vi "AC Couple (1 Ch DBL Array).vi"(8 "error in (no error)":errorcluster, 10 "Signal":dbl[](array[numeric])) -> (0 "error out":errorcluster, 1 "DC":dbl, 2 "AC Coupled":dbl[](array[numeric]))   [LabVIEW 2017, in "VibrationAnalysisFunctions.lvlib"]
uses:
  <vilib>/addons/InsightCM/Utilities/Analysis/Vibration/VibrationAnalysisFunctions.lvlib
  <vilib>/Analysis/baseanly.llb/Mean (DBL).vi
  <vilib>/Analysis/0measdsp.llb/Scaled Time Domain Window (DBL).vi
  <vilib>/Analysis/NI_AALPro.lvlib
  <vilib>/Analysis/NI_AALBase.lvlib
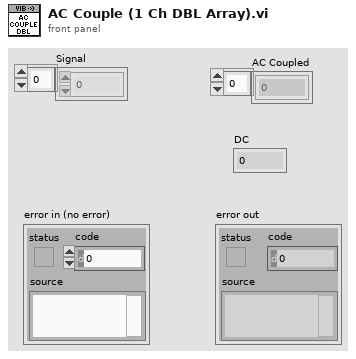
[diagram p1: front panel]
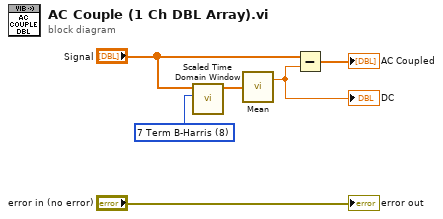
[diagram p0: block diagram]
diagram:
  w4 = u16 8 items=["None ", "Hanning", "Hamming", "Blackman-Harris", "Exact Blackman", "Blackman", "Flat Top", "4 Term B-Harris ", "7 Term B-Harris", "Low Sidelobe"] ("window")
  n1 = call-poly <vilib>:"Scaled Time Domain Window.vi"("window"=w4, "X"="Signal") -> ("Windowed X"=w3:dbl[])  [unwired: 7 in, 2 out]
  n2 = call-poly <vilib>:"Mean.vi"("X"=w3) -> ("mean"=w2:dbl)  [unwired: 1 out]
  "DC" <- w2
  n3 = Subtract(x="Signal", y=w2) -> (x-y=→"AC Coupled":dbl[])
  "error out" <- "error in (no error)"
